vi "Clear Reference.vi"(8 "error in (no error)":errorcluster, 11 "VI Reference Control in":refnum<class "VI Reference Control.lvclass">) -> (0 "error out":errorcluster, 3 "VI Reference Control out":refnum<class "VI Reference Control.lvclass">)   [LabVIEW 2016, in "VI Reference Control.lvclass"]
uses:
  VI Reference Control.lvclass
  VI Reference Control.lvclass/VI Reference Control.ctl
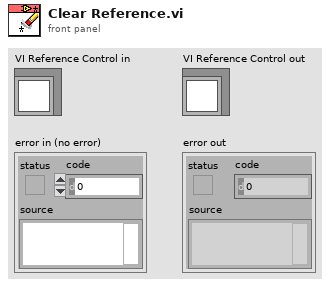
[diagram p1: front panel]
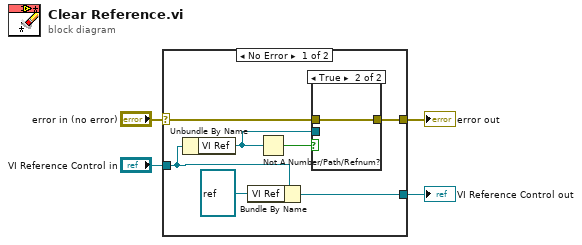
[diagram p0: block diagram]
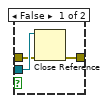
[diagram p2: hidden frame]
diagram:
  n1 = case shown="No Error" "error in (no error)" {
    selector: "error in (no error)" -> [w9 w17]
    tunnel: [w8 w17] -> w3
    tunnel: [w6 w16] -> w1
    tunnel: "VI Reference Control in" -> [w7 w16]
    frame No Error {
      n2 = Unbundle By Name(w7) -> ("VI Ref"=w10:refnum<vi>)
      n3 = Bundle By Name(cluster=w7, "VI Ref"=refnum<vi> refnum) -> (w6:refnum<class "VI Reference Control.lvclass">)
      n4 = Not A Number/Path/Refnum?(number/path/refnum=w10) -> (NaN/Path/Refnum?=w11:bool)
      n5 = case shown="True" w11 {
        tunnel: w10 -> [w14 _]
        tunnel: w9 -> [w13 w15]
        tunnel: [w12 w15] -> w8
        frame False {
          n6 = Close Reference(reference=w14, error in (no error)=w13) -> (error out=w12:errorcluster)
        }
        frame True {
        }
      }
    }
    frame Error {
    }
  }
  "error out" <- w3
  "VI Reference Control out" <- w1
